vi "CTRE_SensoredTank_Set.vi"(8 "Turn":dbl, 9 "Forward":dbl, 10 "Talon SRX Control Mode":T7, 11 "Sensored Tank":T1={"Sensored Gearbox Left"={"Smart Motor Controller"={"DeviceStatus"={"status"=FALSE, "code"=0, "source"=""}, "Type"=enum."PWM", "PWM"={"PWM Channel"=enum."PWM 1", "DeadBand"={"Name"="", "maxPositivePwm"=0, "minPositivePwm"=0, "centerPwm"=0, "maxNegativePwm"=0, "minNegativePwm"=0, "angularRange"=0}}, "CAN"={"Device Number"=0, "SetOutput VI Ref"=variant(enum8{"Percent VBus", "Current", "Speed", "Position", "Voltage"} enum."Percent VBus"), "GetOutput VI Ref"=variant(refnum<k1> refnum), "Enable VI Ref"=variant(dbl 12.0), "Disable VI Ref"=variant(enum8{"Percent VBus", "Speed", "Position", "Slave", "Unchanged / Invalid", "Voltage Compensation", "Current", "Motion Profile"} enum."Percent VBus"), "Data"=variant}, "Invert"=FALSE}, "Invert"=FALSE, "Gear Ratio"=0.0}, "Sensored Gearbox Right "={"Smart Motor Controller"={"DeviceStatus"={"status"=FALSE, "code"=0, "source"=""}, "Type"=enum."PWM", "PWM"={"PWM Channel"=enum."PWM 1", "DeadBand"={"Name"="", "maxPositivePwm"=0, "minPositivePwm"=0, "centerPwm"=0, "maxNegativePwm"=0, "minNegativePwm"=0, "angularRange"=0}}, "CAN"={"Device Number"=0, "SetOutput VI Ref"=variant(enum8{"Percent VBus", "Current", "Speed", "Position", "Voltage"} enum."Percent VBus"), "GetOutput VI Ref"=variant(refnum<k1> refnum), "Enable VI Ref"=variant(dbl 12.0), "Disable VI Ref"=variant(enum8{"Percent VBus", "Speed", "Position", "Slave", "Unchanged / Invalid", "Voltage Compensation", "Current", "Motion Profile"} enum."Percent VBus"), "Data"=variant}, "Invert"=FALSE}, "Invert"=FALSE, "Gear Ratio"=0.0}, "Wheel Radius"=0.0, "Distance Between Wheels"=0.0}) -> (2 "SmartTank":T8, 3 "Sensored Tank":T1={"Sensored Gearbox Left"={"Smart Motor Controller"={"DeviceStatus"={"status"=FALSE, "code"=0, "source"=""}, "Type"=enum."PWM", "PWM"={"PWM Channel"=enum."PWM 1", "DeadBand"={"Name"="", "maxPositivePwm"=0, "minPositivePwm"=0, "centerPwm"=0, "maxNegativePwm"=0, "minNegativePwm"=0, "angularRange"=0}}, "CAN"={"Device Number"=0, "SetOutput VI Ref"=variant(enum8{"Percent VBus", "Current", "Speed", "Position", "Voltage"} enum."Percent VBus"), "GetOutput VI Ref"=variant(refnum<k1> refnum), "Enable VI Ref"=variant(dbl 12.0), "Disable VI Ref"=variant(enum8{"Percent VBus", "Speed", "Position", "Slave", "Unchanged / Invalid", "Voltage Compensation", "Current", "Motion Profile"} enum."Percent VBus"), "Data"=variant}, "Invert"=FALSE}, "Invert"=FALSE, "Gear Ratio"=0.0}, "Sensored Gearbox Right "={"Smart Motor Controller"={"DeviceStatus"={"status"=FALSE, "code"=0, "source"=""}, "Type"=enum."PWM", "PWM"={"PWM Channel"=enum."PWM 1", "DeadBand"={"Name"="", "maxPositivePwm"=0, "minPositivePwm"=0, "centerPwm"=0, "maxNegativePwm"=0, "minNegativePwm"=0, "angularRange"=0}}, "CAN"={"Device Number"=0, "SetOutput VI Ref"=variant(enum8{"Percent VBus", "Current", "Speed", "Position", "Voltage"} enum."Percent VBus"), "GetOutput VI Ref"=variant(refnum<k1> refnum), "Enable VI Ref"=variant(dbl 12.0), "Disable VI Ref"=variant(enum8{"Percent VBus", "Speed", "Position", "Slave", "Unchanged / Invalid", "Voltage Compensation", "Current", "Motion Profile"} enum."Percent VBus"), "Data"=variant}, "Invert"=FALSE}, "Invert"=FALSE, "Gear Ratio"=0.0}, "Wheel Radius"=0.0, "Distance Between Wheels"=0.0})   [LabVIEW 2016]
uses:
  <vilib>/Rock Robotics/WPI/ThirdParty/CanMotor/CTRLib-LV-TalonSRX/Framework/SensoredTank.ctl
  <vilib>/Rock Robotics/WPI/ThirdParty/CanMotor/CTRLib-LV-TalonSRX/Framework/SensoredGearbox.ctl
  <vilib>/Rock Robotics/WPI/MotorControl/WPI_MotorControlDeviceRef.ctl
  <vilib>/Rock Robotics/WPI/MotorControl/WPI_MotorControlType.ctl
  <vilib>/Rock Robotics/SystemInterfaces/DIO/FPGA_DIOPWMChannel.ctl
  <vilib>/Rock Robotics/WPI/PWM/WPI_PWMDeadband.ctl
  <vilib>/Rock Robotics/WPI/ThirdParty/CanMotor/CTRLib-LV-TalonSRX/CTRE_CANTalonSRX_ControlMode.ctl
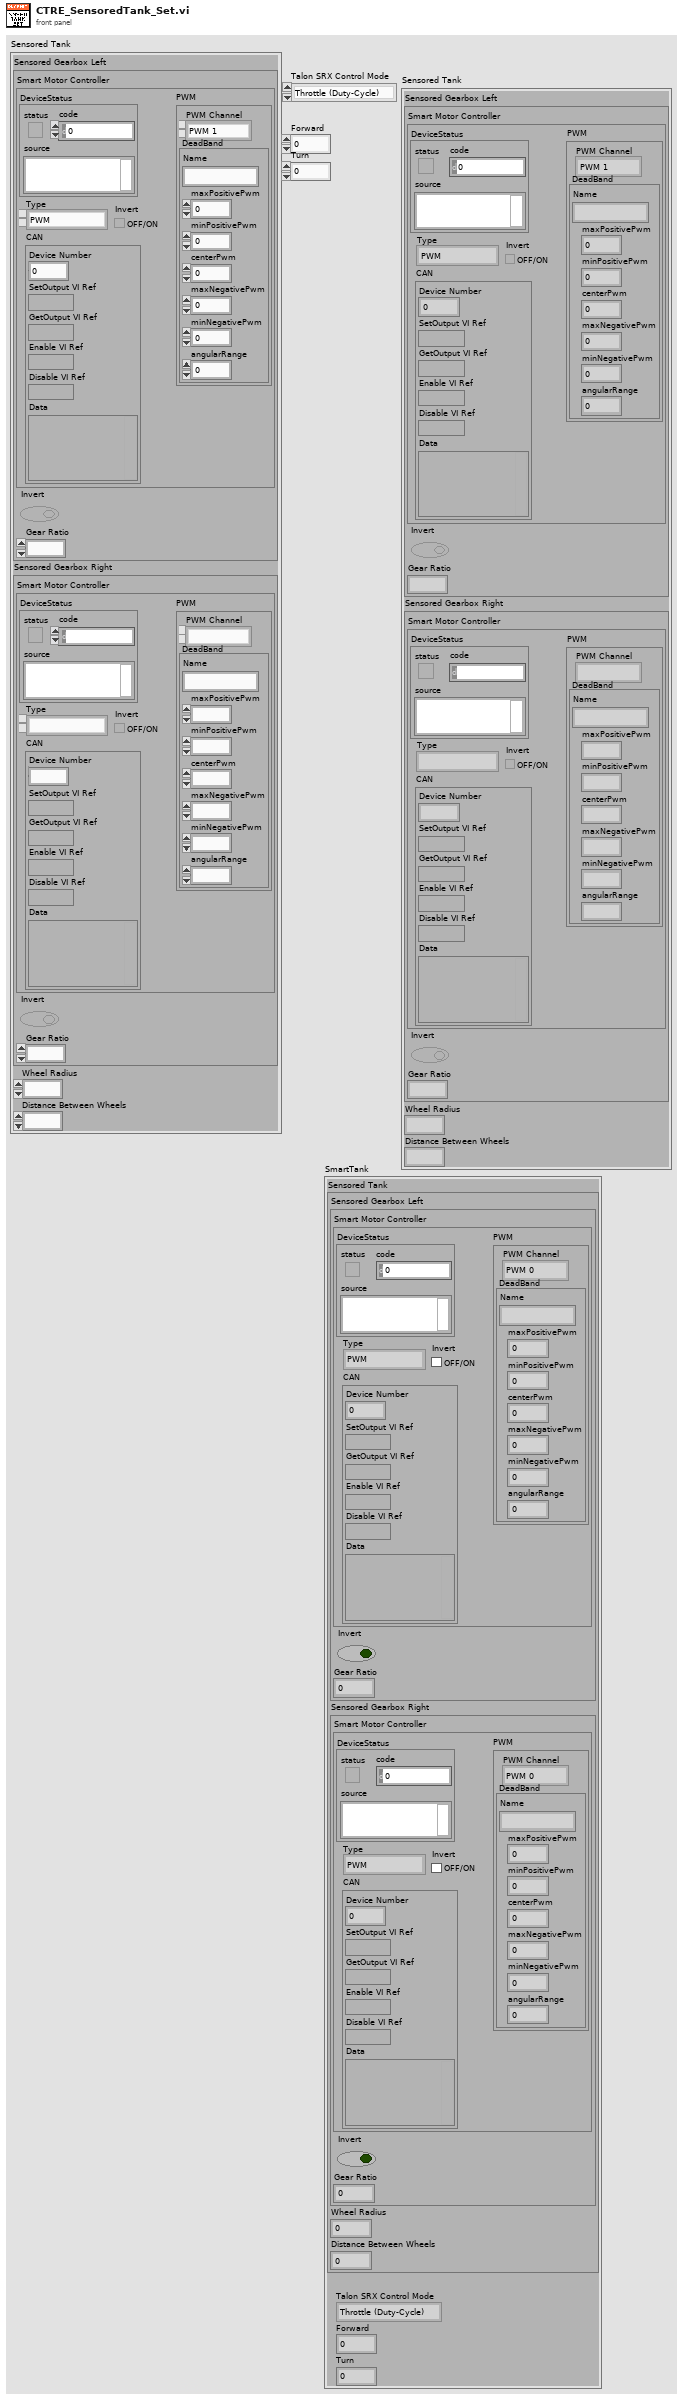
[diagram p1: front panel]
types:
  T1 = typedef "SensoredTank.ctl" = cluster{"Sensored Gearbox Left":T2, "Sensored Gearbox Right ":T2, "Wheel Radius":dbl, "Distance Between Wheels":dbl}
  T2 = typedef "SensoredGearbox.ctl" = cluster{"Smart Motor Controller":T3, "Invert":bool, "Gear Ratio":dbl}
  T3 = typedef "WPI_MotorControlDeviceRef.ctl" = cluster{"DeviceStatus":errorcluster, "Type":T4, "PWM":cluster{"PWM Channel":T5, "DeadBand":T6}, "CAN":cluster{"Device Number":u8, "SetOutput VI Ref":variant, "GetOutput VI Ref":variant, "Enable VI Ref":variant, "Disable VI Ref":variant, "Data":variant}, "Invert":bool}
  T4 = typedef "WPI_MotorControlType.ctl" = enum16{"PWM", "CAN"}
  T5 = typedef "FPGA_DIOPWMChannel.ctl" = enum8{"PWM 0", "PWM 1", "PWM 2", "PWM 3", "PWM 4", "PWM 5", "PWM 6", "PWM 7", "PWM 8", "PWM 9", "PWM MXP 0", "PWM MXP 1", "PWM MXP 2", "PWM MXP 3", "PWM MXP 4", "PWM MXP 5", "PWM MXP 6", "PWM MXP 7", "PWM MXP 8", "PWM MXP 9", "Invalid"}
  T6 = typedef "WPI_PWMDeadband.ctl" = cluster{"Name":string, "maxPositivePwm":i32, "minPositivePwm":i32, "centerPwm":i32, "maxNegativePwm":i32, "minNegativePwm":i32, "angularRange":u16}
  T7 = typedef "CTRE_CANTalonSRX_ControlMode.ctl" = enum16{"Throttle (Duty-Cycle)", "Position Closed-Loop", "Velocity Closed-Loop", "Current Closed-Loop", "Voltage Compensation", "Slave Follower", "Motion Profile", "Motion Magic"}
  T8 = cluster{"Sensored Tank":T1, "Talon SRX Control Mode":T7, "Forward":dbl, "Turn":dbl}
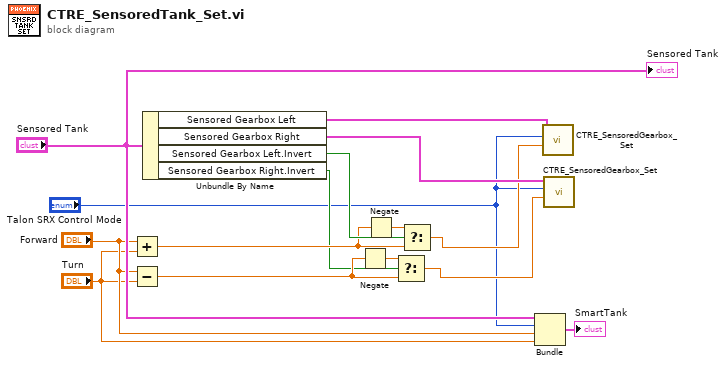
[diagram p0: block diagram]
diagram:
  n1 = Add(x="Forward", y="Turn") -> (x+y=w10:dbl)
  n2 = Subtract(x="Forward", y="Turn") -> (x-y=w8:dbl)
  n3 = Unbundle By Name("Sensored Tank") -> ("Sensored Gearbox Left"=w15:T2, "Sensored Gearbox Right"=w14:T2, "Sensored Gearbox Left.Invert"=w13:bool, "Sensored Gearbox Right.Invert"=w6:bool)
  n4 = Negate(x=w8) -> (-x=w9:dbl)
  n5 = Negate(x=w10) -> (-x=w11:dbl)
  n6 = Select(t=w9, s=w6, f=w8) -> (s? t:f=w7:dbl)
  n7 = Select(t=w11, s=w13, f=w10) -> (s? t:f=w12:dbl)
  n8 = Bundle("Sensored Tank"="Sensored Tank", "Talon SRX Control Mode"="Talon SRX Control Mode", "Forward"="Forward", "Turn"="Turn") -> (→"SmartTank":T8)  [unwired: 1 in]
  n9 = call <vilib>:"CTRE_SensoredGearbox_Set.vi"("Output"=w12, "Talon SRX Control Mode"="Talon SRX Control Mode", "Sensored Gearbox"=w15) -> ()  [unwired: 8 in, 1 out]
  n10 = call <vilib>:"CTRE_SensoredGearbox_Set.vi"("Output"=w7, "Talon SRX Control Mode"="Talon SRX Control Mode", "Sensored Gearbox"=w14) -> ()  [unwired: 8 in, 1 out]
  "Sensored Tank" <- "Sensored Tank"
